vi "DataReadingStringToClusterFormar.vi"(11 "StringFormat":string[](array[string])) -> (3 "ClusterFormat":T1)   [LabVIEW 2014]
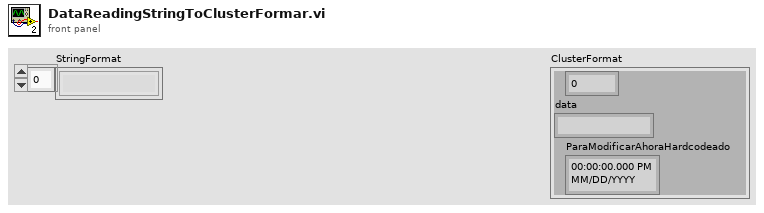
[diagram p1: front panel]
types:
  T1 = cluster{dbl, "data":string, "ParaModificarAhoraHardcodeado":timestamp}
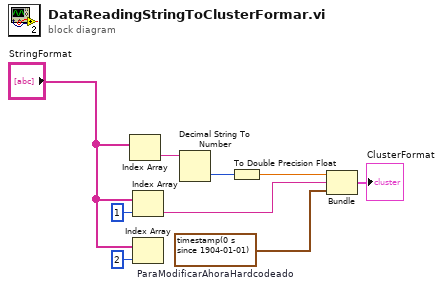
[diagram p0: block diagram]
diagram:
  w3 = timestamp(0 s since 1904-01-01)  # ParaModificarAhoraHardcodeado
  n1 = Index Array(array="StringFormat") -> (element=w9:string)  [unwired: 1 in]
  n2 = Index Array(array="StringFormat", index=1) -> (element=w6:string)
  n3 = Index Array(array="StringFormat", index=2) -> ()  [unwired: 1 out]
  n4 = Decimal String To Number(string=w9) -> (number=w5:i32)  [unwired: 2 in, 1 out]
  n5 = To Double Precision Float(number=w5) -> (double precision float=w4:dbl)
  n6 = Bundle(w4, "data"=w6, "ParaModificarAhoraHardcodeado"=w3) -> (→"ClusterFormat":T1)  [unwired: 1 in]
